vi "Lickometer-Read.vi"(7 "Device reference":refnum<vi>, 8 "error in (no error)":errorcluster) -> (0 "error out":errorcluster, 1 "Lick start?":bool, 3 "Lick?":bool)   [LabVIEW 2015]
doc: "Reads a lickometer.\n\nDevice reference: which lickometer to read?\nLick?: Is a lick port being licked?\nLick start?: Is a lick starting?\n\nDebouncing is only done on the ON transitions, and consists of requiring the signal to be stable high for some amount of time (specified in the lickometer settings) before considering it ON."
uses:
  Typedefs/Lickometer.ctl
  Rack/Typedefs/OutputRequest refnum.ctl
  Rack/Typedefs/OutputRequest.ctl
  Rack/Typedefs/InputData cluster.ctl
  Rack/Methods/Port drivers/DigitalInput-DataCluster.ctl
panel:
  out "Lickometer":T1={"Settings"={"Min lick duration"=0, "Port name"="", "Port index"=-1}, "Lick"=FALSE, "Debouncing"={"Semaphore"=refnum, "Lick start"=0}, "OutputRequest event ref"=refnum, "InputData reference"=refnum, "Active hi?"=FALSE}
  # "Just a local copy for convenience"
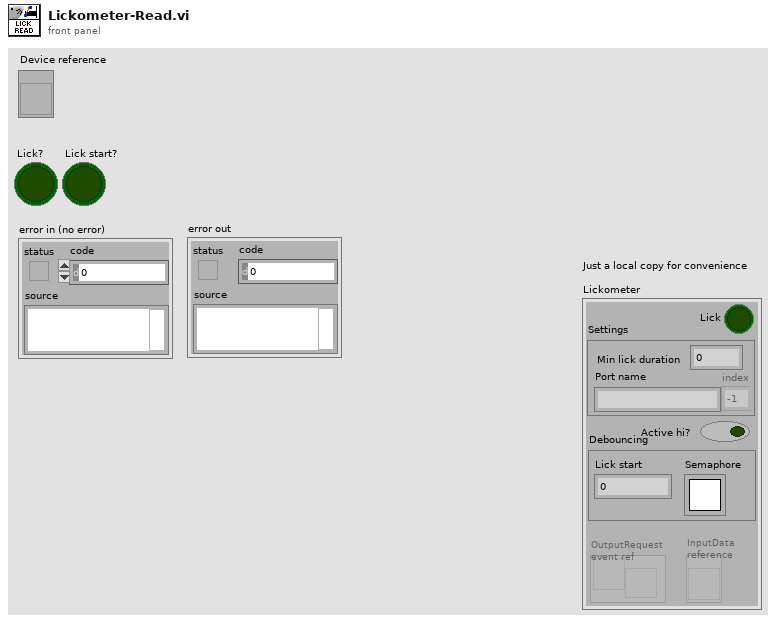
[diagram p1: front panel]
types:
  T1 = typedef "Lickometer.ctl" = cluster{"Settings":cluster{"Min lick duration":u32, "Port name":string, "Port index":i32}, "Lick":bool, "Debouncing":cluster{"Semaphore":T2, "Lick start":u32}, "OutputRequest event ref":T3, "InputData reference":refnum<vi>, "Active hi?":bool}
  T2 = typedef "Semaphore RefNum" = refnum<k1>
  T3 = typedef "OutputRequest refnum.ctl" = refnum<user-event>
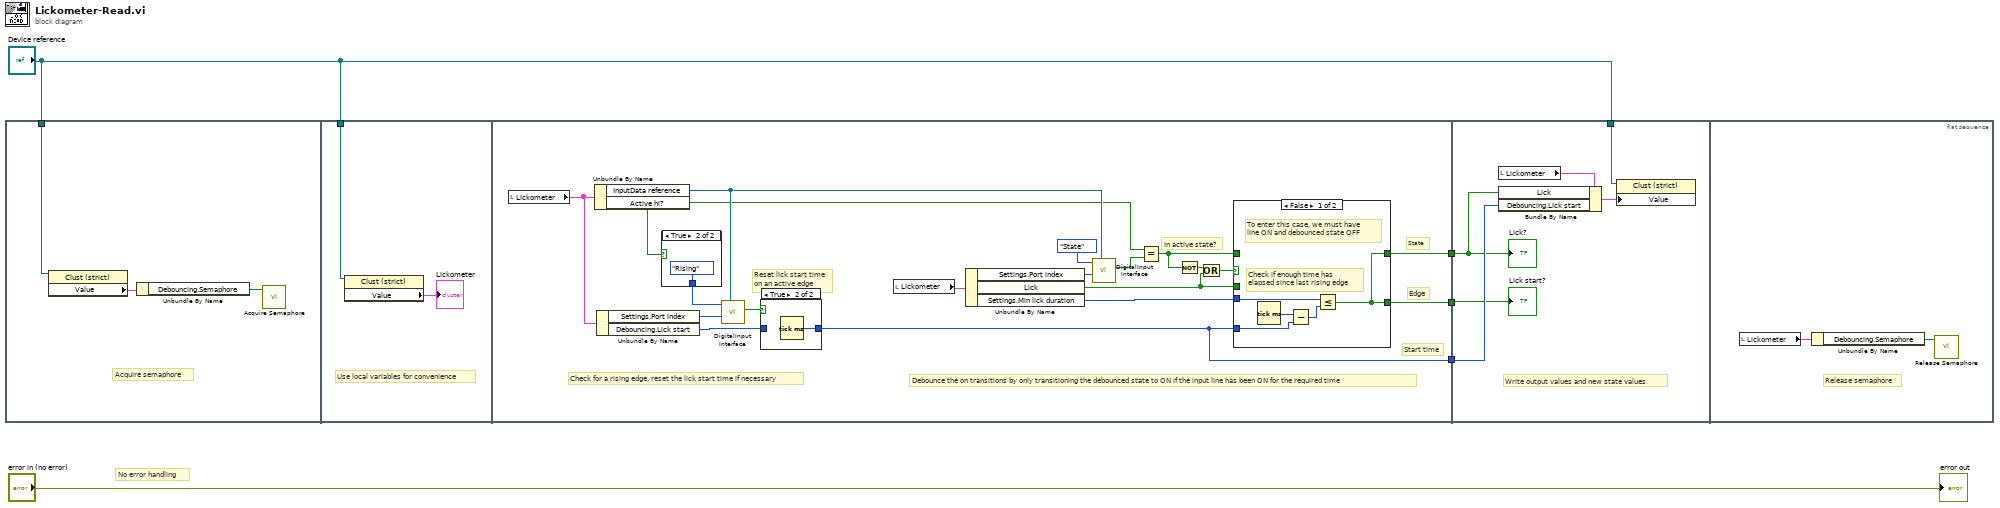
[diagram p0: block diagram]
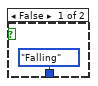
[diagram p2: hidden frame]
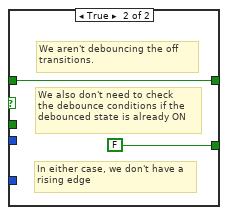
[diagram p3: hidden frame]
diagram:
  # "No error handling"
  n1 = flat-sequence {
    tunnel: "Device reference" -> [w8]
    tunnel: "Device reference" -> [w9]
    tunnel: [w18] -> w5
    tunnel: [w17] -> w4
    tunnel: [w16] -> w3
    tunnel: w5 -> [w45]
    tunnel: w4 -> [w43]
    tunnel: w3 -> [w44]
    tunnel: "Device reference" -> [w41]
    frame #0 {
      # "Acquire semaphore"
      n2 = property class="Clust (strict)"(reference=w8) -> ("Value"=w7:T1)  [unwired: 1 in, 2 out]
      n3 = Unbundle By Name(w7) -> ("Debouncing.Semaphore"=w6:T2)
      n4 = call <vilib>:"Acquire Semaphore.vi"("semaphore"=w6) -> ()  [unwired: 4 in, 3 out]
    }
    frame #1 {
      # "Use local variables for convenience"
      n5 = property class="Clust (strict)"(reference=w9) -> ("Value"=→"Lickometer":T1)  [unwired: 1 in, 2 out]
    }
    frame #2 {
      # "In active state?"
      # "Reset lick start time\non an active edge"
      # "Start time"
      # "Edge"
      # "State"
      # "Debounce the on transitions by only transitioning the debounced state to ON if the input line has been ON for the required time"
      # "Check for a rising edge, reset the lick start time if necessary"
      n6 = local read "Lickometer"() -> (w15:T1)
      n7 = Unbundle By Name(w15) -> ("InputData reference"=w14:refnum<vi>, "Active hi?"=w11:bool)
      n8 = Unbundle By Name(w15) -> ("Settings.Port index"=w29:i32, "Debouncing.Lick start"=w28:u32)
      n9 = case shown="True" w11 {
        tunnel: [enum16{"State", "Rising", "Falling"}."Falling" ("Data type") enum16{"State", "Rising", "Falling"}."Rising" ("Data type")] -> w27
        frame False {
        }
        frame True {
        }
      }
      n10 = call "DigitalInput Interface.vi"("InputData Refnum"=w14, "Port index"=w29, "Data type"=w27) -> ("Data"=w26:bool)  [unwired: 8 in]
      n11 = case shown="True" w26 {
        tunnel: w28 -> [w39 _]
        tunnel: [w39 w40] -> w18
        frame False {
        }
        frame True {
          n12 = Tick Count (ms)() -> (millisecond timer value=w40:u32)
        }
      }
      n13 = local read "Lickometer"() -> (w24:T1)
      n14 = Unbundle By Name(w24) -> ("Settings.Port index"=w23:i32, "Lick"=w20:bool, "Settings.Min lick duration"=w22:u32)
      n15 = call "DigitalInput Interface.vi"("InputData Refnum"=w14, "Port index"=w23, "Data type"=enum16{"State", "Rising", "Falling"}."State") -> ("Data"=w13:bool)  [unwired: 8 in]
      n16 = Equal?(x=w11, y=w13) -> (x = y?=w12:bool)
      n17 = Not(x=w12) -> (.not. x?=w21:bool)
      n18 = Or(x=w21, y=w20) -> (x .or. y?=w19:bool)
      n19 = case shown="False" w19 {
        tunnel: w20 -> [_ _]
        tunnel: w22 -> [w34 _]
        tunnel: w18 -> [w33 _]
        tunnel: w12 -> [_ w38]
        tunnel: [w32 w38] -> w16
        tunnel: [w32 FALSE] -> w17
        frame False {
          # "To enter this case, we must have\nline ON and debounced state OFF"
          # "Check if enough time has\nelapsed since last rising edge"
          n20 = Tick Count (ms)() -> (millisecond timer value=w36:u32)
          n21 = Subtract(x=w36, y=w33) -> (x-y=w35:u32)
          n22 = Less Or Equal?(x=w34, y=w35) -> (x <= y?=w32:bool)
        }
        frame True {
          # "In either case, we don't have a\nrising edge"
          # "We also don't need to check\nthe debounce conditions if the\ndebounced state is already ON"
          # "We aren't debouncing the off \ntransitions."
        }
      }
    }
    frame #3 {
      # "Write output values and new state values"
      n23 = local read "Lickometer"() -> (w46:T1)
      n24 = Bundle By Name(cluster=w46, "Lick"=w44, "Debouncing.Lick start"=w45) -> (w42:T1)
      n25 = property class="Clust (strict)"(reference=w41, "Value"=w42) -> ()  [unwired: 1 in, 2 out]
      "Lick?" <- w44
      "Lick start?" <- w43
    }
    frame #4 {
      # "Release semaphore"
      n26 = local read "Lickometer"() -> (w47:T1)
      n27 = Unbundle By Name(w47) -> ("Debouncing.Semaphore"=w48:T2)
      n28 = call <vilib>:"Release Semaphore.vi"("semaphore"=w48) -> ()  [unwired: 5 in, 2 out]
    }
  }
  "error out" <- "error in (no error)"
